vi "Pressure device cluster to String.vi"(11 "Temperature Device Settings":T1) -> (3 "Data to send":string="EXCT:TYPE:Unipolar:MAG:10.00:EXCT:NICK:MB1.T1:LOOP:AUX:None:PSET:1.0:HTR:None:ISET:1.0:HAUT:Manual:HSET:0.0:PIDT:Manual:DSET:1.0:TSET:0K:LVL:MB1.T1:LOOP:MAN:HVER:0:FVER:20.6:SERL:102750119:MAN:CAL:OFFS:0.0000:COLD:1.0000:INT:Linear:SCAL:1.0000:FILE:RP5.DAT:HOTL:1023.1500:CAL:TYPE:PTC:SIG:VOLT:1405.9mV:CURR:10µA:TEMP:1023.15K:POWR:14.059µW:RES:140590?:SLOP:137.409?/K:FLOW:NOT_FOUND:SIG:TEMP\n")   [LabVIEW 2013, in "Mercury iXX.lvlib" / "Pressure.lvlib"]
uses:
  <instrlib>/Mercury iXX/Public/Libraries/Pressure.lvlib
  <instrlib>/Mercury iXX/Public/Libraries/Pressure/Controls/Pressure Device (Set).ctl
  <instrlib>/Mercury iXX/Public/Libraries/Pressure/Controls/Pressure Sensor Type.ctl
  <instrlib>/Mercury iXX/Public/Libraries/Pressure/Controls/Calibration Cluster.ctl
  <instrlib>/Mercury iXX/Public/Libraries/Pressure/Controls/Calibration Interpolation.ctl
  <instrlib>/Mercury iXX/Public/Libraries/Pressure/Controls/Loop Cluster.ctl
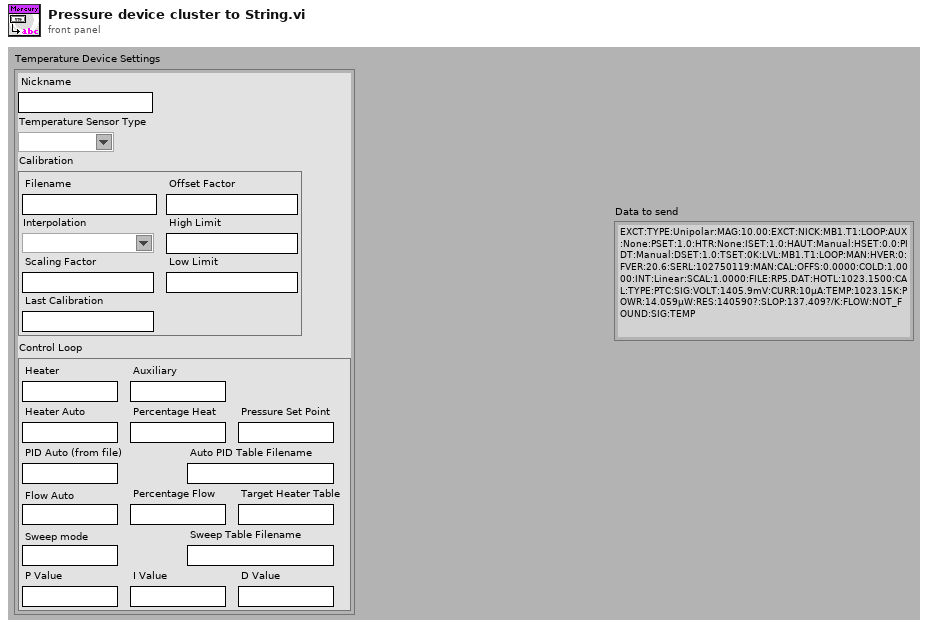
[diagram p1: front panel]
types:
  T1 = typedef "Mercury iXX.lvlib/Pressure.lvlib/Pressure Device (Set).ctl" = cluster{"Nickname":string, "Temperature Sensor Type":T2, "Calibration":T3, "Control Loop":T5}
  T2 = typedef "Mercury iXX.lvlib/Pressure.lvlib/Pressure Sensor Type.ctl" = string
  T3 = typedef "Mercury iXX.lvlib/Pressure.lvlib/Calibration Cluster.ctl" = cluster{"Filename":string, "Interpolation":T4, "Scaling Factor":string, "Offset Factor":string, "High Limit":string, "Low Limit":string, "Last Calibration":string}
  T4 = typedef "Mercury iXX.lvlib/Pressure.lvlib/Calibration Interpolation.ctl" = string
  T5 = typedef "Mercury iXX.lvlib/Pressure.lvlib/Loop Cluster.ctl" = cluster{"Heater":string, "Auxiliary":string, "Heater Auto":string, "Percentage Heat":string, "Pressure Set Point":string, "PID Auto (from file)":string, "P Value":string, "I Value":string, "D Value":string, "Auto PID Table Filename":string, "Flow Auto":string, "Target Heater Table":string, "Sweep mode":string, "Sweep Table Filename":string, "Percentage Flow":string}
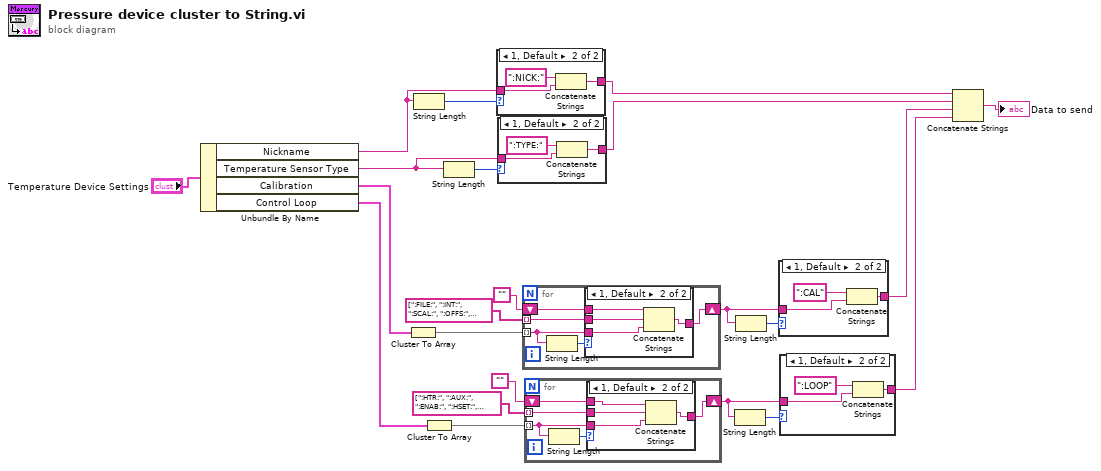
[diagram p0: block diagram]
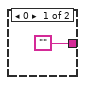
[diagram p2: hidden frame]
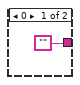
[diagram p3: hidden frame]
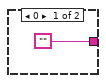
[diagram p6: hidden frame]
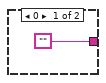
[diagram p7: hidden frame]
diagram:
  n1 = Unbundle By Name("Temperature Device Settings") -> ("Nickname"=w18:string, "Temperature Sensor Type"=w16:T2, "Calibration"=w21:T3, "Control Loop"=w20:T5)
  n2 = Cluster To Array(cluster=w21) -> (array=w11:T4[])
  n3 = String Length(string=w18) -> (length=w19:i32)
  n4 = Cluster To Array(cluster=w20) -> (array=w9:string[])
  n5 = String Length(string=w16) -> (length=w17:i32)
  n6 = case shown="1, Default" w19 {
    tunnel: w18 -> [_ w25]
    tunnel: ["" w26] -> w15
    frame 0 {
    }
    frame 1, Default {
      n7 = Concatenate Strings(":NICK:" ("string"), w25) -> (w26:string)
    }
  }
  n8 = case shown="1, Default" w17 {
    tunnel: w16 -> [_ w29]
    tunnel: ["" w30] -> w14
    frame 0 {
    }
    frame 1, Default {
      n9 = Concatenate Strings(":TYPE:" ("string"), w29) -> (w30:string)
    }
  }
  n10 = for {
    tunnel: w11 -> [w34] mode=indexing
    tunnel: string[] [":FILE:", ":INT:", ":SCAL:", ":OFFS:", ":HOTL:", ":COLDL:"] ("Excitation") -> [w33] mode=indexing
    shift-right: [w32] -> w4
    shift-left: "" -> [w31]
    n11 = String Length(string=w34) -> (length=w35:i32)
    n12 = case shown="1, Default" w35 {
      tunnel: w34 -> [_ w39]
      tunnel: [w36 w40] -> w32
      tunnel: w33 -> [_ w38]
      tunnel: w31 -> [w36 w37]
      frame 0 {
      }
      frame 1, Default {
        n13 = Concatenate Strings(w37, w38, w39) -> (w40:string)
      }
    }
  }
  n14 = for {
    tunnel: w9 -> [w44] mode=indexing
    tunnel: string[] [":HTR:", ":AUX:", ":ENAB:", ":HSET:", ":TSET:", ":PIDT:", ":P:", ":I:", ":D:", ":PIDF:", ":FAUT:", ":THTF:", ":SWMD:", ":SWFL:", ":FSET:"] ("Excitation") -> [w43] mode=indexing
    shift-right: [w42] -> w3
    shift-left: "" -> [w41]
    n15 = String Length(string=w44) -> (length=w45:i32)
    n16 = case shown="1, Default" w45 {
      tunnel: w44 -> [_ w49]
      tunnel: [w46 w50] -> w42
      tunnel: w43 -> [_ w48]
      tunnel: w41 -> [w46 w47]
      frame 0 {
      }
      frame 1, Default {
        n17 = Concatenate Strings(w47, w48, w49) -> (w50:string)
      }
    }
  }
  n18 = String Length(string=w3) -> (length=w1:i32)
  n19 = String Length(string=w4) -> (length=w2:i32)
  n20 = case shown="1, Default" w2 {
    tunnel: ["" w54] -> w8
    tunnel: w4 -> [_ w53]
    frame 0 {
    }
    frame 1, Default {
      n21 = Concatenate Strings(":CAL" ("string"), w53) -> (w54:string)
    }
  }
  n22 = case shown="1, Default" w1 {
    tunnel: ["" w58] -> w7
    tunnel: w3 -> [_ w57]
    frame 0 {
    }
    frame 1, Default {
      n23 = Concatenate Strings(":LOOP" ("string"), w57) -> (w58:string)
    }
  }
  n24 = Concatenate Strings(w15, w14, w8, w7) -> (→"Data to send":string)
